vi "SSL_CTX_load_certificate.vi"(8 "error in (no error)":errorcluster, 9 "cert path":T1, 10 "CTX":i32, 11 "path in":path) -> (0 "error out":errorcluster, 2 "CTX":i32, 3 "path out":path)   [LabVIEW 2018, in "AWS_IoT.lvlib"]
doc: "Load client cert, client key, and CA file into SSL_CTX\n\nMIT License\n\nCopyright (c) 2016 Indie-Energy\n\nPermission is hereby granted, free of charge, to any person obtaining a copy\nof this software and associated documentation files (the \"Software\"), to deal\nin the Software without restriction, including without limitation the rights\nto use, copy, modify, merge, publish, distribute, sublicense, and/or sell\ncopies of the Software, and to permit persons to whom the Software is\nfurnished to do so, subject to the following conditions:\n\nThe above copyright notice and this permission notice shall be included in all\ncopies or substantial portions of the Software.\n\nTHE SOFTWARE IS PROVIDED \"AS IS\", WITHOUT WARRANTY OF ANY KIND, EXPRESS OR\nIMPLIED, INCLUDING BUT NOT LIMITED TO THE WARRANTIES OF MERCHANTABILITY,\nFITNESS FOR A PARTICULAR PURPOSE AND NONINFRINGEMENT. IN NO EVENT SHALL THE\nAUTHORS OR COPYRIGHT HOLDERS BE LIABLE FOR ANY CLAIM, DAMAGES OR OTHER\nLIABILITY, WHETHER IN AN ACTION OF CONTRACT, TORT OR OTHERWISE, ARISING FROM,\nOUT OF OR IN CONNECTION WITH THE SOFTWARE OR THE USE OR OTHER DEALINGS IN THE\nSOFTWARE."
uses:
  AWS_IoT.lvlib
  Controls/certs.ctl
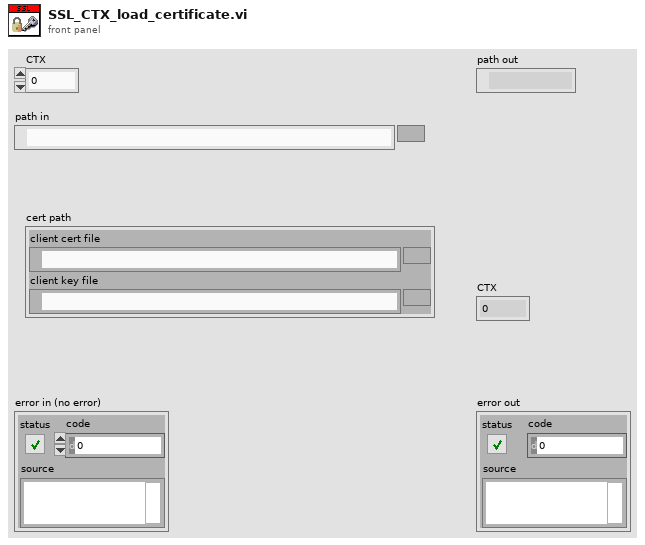
[diagram p1: front panel]
types:
  T1 = typedef "AWS_IoT.lvlib/certs.ctl" = cluster{"client cert file":path, "client key file":path}
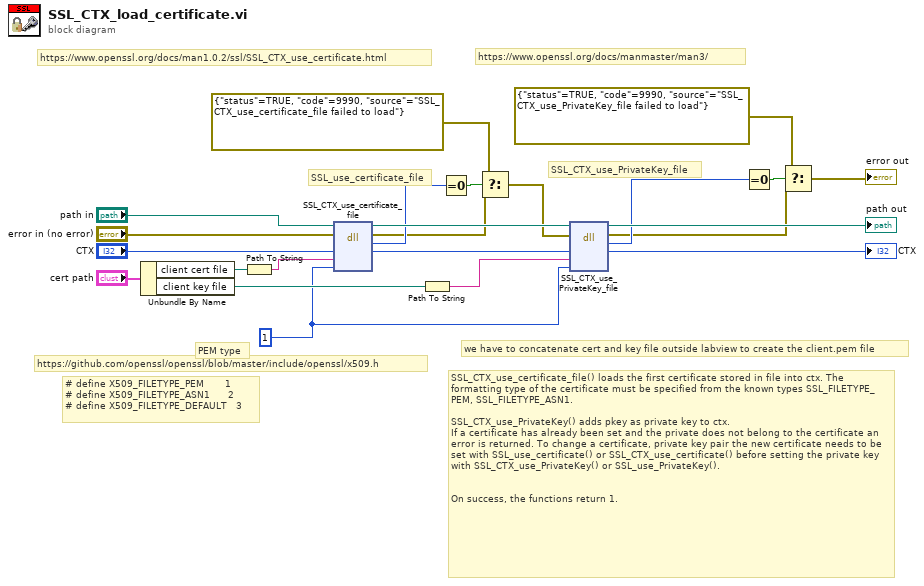
[diagram p0: block diagram]
diagram:
  w20 = 1 ("type")
  # "we have to concatenate cert and key file outside labview to create the client.pem file"
  # "https://github.com/openssl/openssl/blob/master/include/openssl/x509.h"
  # "https://www.openssl.org/docs/man1.0.2/ssl/SSL_CTX_use_certificate.html"
  # "https://www.openssl.org/docs/manmaster/man3/"
  # "SSL_CTX_use_certificate_file() loads the first certificate stored in file into ctx. The formatting type of the certificate must be specified from the known types SSL_FILETYPE_PEM, SSL_FILETYPE_ASN1.\n\nSSL_CTX_use_PrivateKey() adds pkey as private key to ctx.  \nIf a certificate has already been set and the private does not belong to the certificate an error is returned. To change a certificate, private key pair the new certificate needs to be set with SSL_use_certificate() or SSL_CTX_use_certificate() before setting the private key with SSL_CTX_use_PrivateKey() or SSL_use_PrivateKey().\n\n\nOn success, the functions return 1."
  # "# define X509_FILETYPE_PEM       1\n# define X509_FILETYPE_ASN1      2\n# define X509_FILETYPE_DEFAULT   3"
  # "SSL_CTX_use_PrivateKey_file"
  # "PEM type"
  # "SSL_use_certificate_file"
  n1 = Unbundle By Name("cert path") -> ("client cert file"=w22:path, "client key file"=w23:path)
  n2 = Path To String(path=w22) -> (string=w19:string)
  n3 = dll-call lib="NIssleay32.*" fn="SSL_CTX_use_certificate_file"(path in="path in", error in="error in (no error)", "CTX"="CTX", "keyfile"=w19, "type"=w20) -> (path out=w15:path, error out=w7:errorcluster, "return type"=w10:i32, "CTX"=w17:i32)  [unwired: 3 in]
  n4 = Path To String(path=w23) -> (string=w13:string)
  n5 = Equal To 0?(x=w10) -> (x = 0?=w9:bool)
  n6 = Select(t=errorcluster {"status"=TRUE, "code"=9990, "source"="SSL_CTX_use_certificate_file failed to load"}, s=w9, f=w7) -> (s? t:f=w6:errorcluster)
  n7 = dll-call lib="NIssleay32.*" fn="SSL_CTX_use_PrivateKey_file"(path in=w15, error in=w6, "CTX"=w17, "keyfile"=w13, "type"=w20) -> (path out=→"path out":path, error out=w2:errorcluster, "return type"=w3:i32, "CTX"=→"CTX":i32)  [unwired: 3 in]
  n8 = Equal To 0?(x=w3) -> (x = 0?=w4:bool)
  n9 = Select(t=errorcluster {"status"=TRUE, "code"=9990, "source"="SSL_CTX_use_PrivateKey_file failed to load"}, s=w4, f=w2) -> (s? t:f=→"error out":errorcluster)
